vi "Boolean array to string of 1s and 0s.vi"(1 "Array":bool[](array[boolean])) -> (0 "String":string)   [LabVIEW 2012]
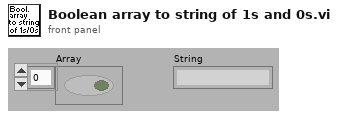
[diagram p1: front panel]
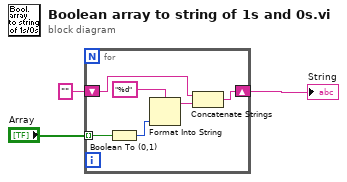
[diagram p0: block diagram]
diagram:
  n1 = for {
    tunnel: "Array" -> [w9] mode=indexing
    shift-right: [w5] -> w2
    shift-left: "" -> [w4]
    n2 = Boolean To (0,1)(Boolean=w9) -> (0, 1=w7:i16)
    n3 = Format Into String(format string="%d", w7) -> (resulting string=w6:string)  [unwired: 2 in, 1 out]
    n4 = Concatenate Strings(w4, w6) -> (w5:string)
  }
  "String" <- w2
